vi "classify error.vi"(8 "error to classify":errorcluster, 11 "testmod runtime in":refnum<class "testmod runtime.lvclass">) -> (0 "classified error":errorcluster, 2 "error classification":T1, 3 "testmod runtime out":refnum<class "testmod runtime.lvclass">)   [LabVIEW 2013, in "testmod runtime.lvclass"]
doc: "Allows a module to classify an error generated at any point during execution. This <b>error classification</b> can then be used by calling code to determine if execution can continue. In addition, this function can be used to allow a component to clear an error, convert an error to a warning, or attempt to recover from an error. Recovery may be attempted only if <b>attempt recovery?</b> is true."
uses:
  testmod runtime.lvclass
  <vilib>/NI/DCAF Module Framework/runtime/error classification.ctl
  <vilib>/NI/DCAF Module Framework/runtime/TBM module execution interface.lvclass
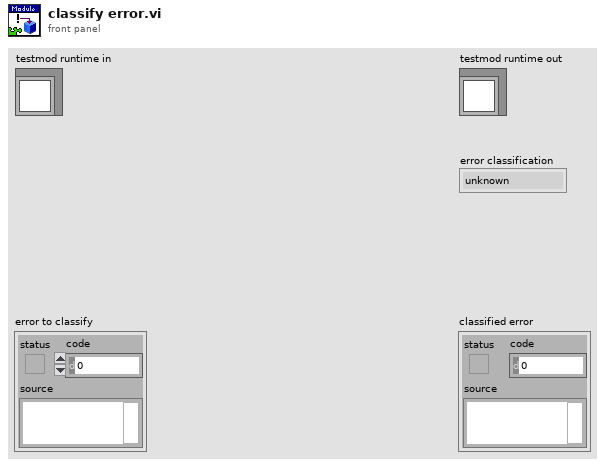
[diagram p1: front panel]
types:
  T1 = typedef "TBM module execution interface.lvclass/error classification.ctl" = enum16{"unknown", "none", "trivial", "recoverable", "critical"}
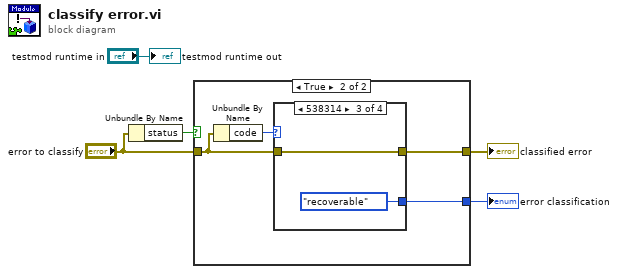
[diagram p0: block diagram]
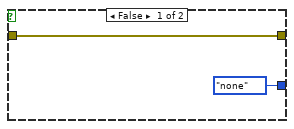
[diagram p2: hidden frame]
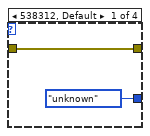
[diagram p3: hidden frame]
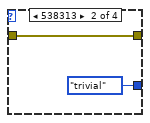
[diagram p4: hidden frame]
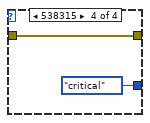
[diagram p5: hidden frame]
diagram:
  n1 = Unbundle By Name("error to classify") -> ("status"=w2:bool)
  n2 = case shown="True" w2 {
    tunnel: [w6 w9] -> w4
    tunnel: [error_classification."none" ("error classification") w10] -> w3
    tunnel: "error to classify" -> [w6 w8]
    frame False {
    }
    frame True {
      n3 = Unbundle By Name(w8) -> ("code"=w11:i32)
      n4 = case shown="538314" w11 {
        tunnel: [error_classification."unknown" ("error classification") error_classification."trivial" ("error classification") error_classification."recoverable" ("error classification") error_classification."critical" ("error classification")] -> w10
        tunnel: w8 -> [w12 w14 w16 w18]
        tunnel: [w12 w14 w16 w18] -> w9
        frame 538312, Default {
        }
        frame 538313 {
        }
        frame 538314 {
        }
        frame 538315 {
        }
      }
    }
  }
  "error classification" <- w3
  "classified error" <- w4
  "testmod runtime out" <- "testmod runtime in"
